vi "Fake Failing Test.vi"() -> ()   [LabVIEW 2017, in "LVUnit Test Executor.Tests.lvlib"]
uses:
  LVUnit Test Executor.Tests.lvlib
panel:
  out "error out":errorcluster={"status"=TRUE, "code"=-1, "source"="Failure"}
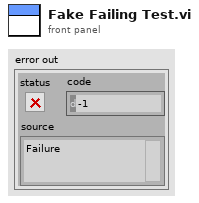
[diagram p1: front panel]
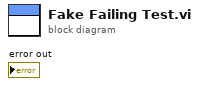
[diagram p0: block diagram]
diagram:
